vi "CCExtractAllDicomInfoFromFile.vi"(8 "error in (no error)":errorcluster, 11 "filename":string) -> (0 "error out":errorcluster, 2 "Values":string[](array[string]), 3 "VariableName":string[](array[string]))   [LabVIEW 2013, in "main.lvlib" / "ClearCanvasLibrary.lvlib"]
uses:
  ClearCanvasLibrary.lvlib
  C:/Users/Simon/SkyDrive/LabView/2013/DM2020/DICOM/ClearCanvasNewBuild/ClearCanvas.Dicom.dll
  ClearCanvasNewBuild/ClearCanvas.Dicom.dll
panel:
  out "Dump":string
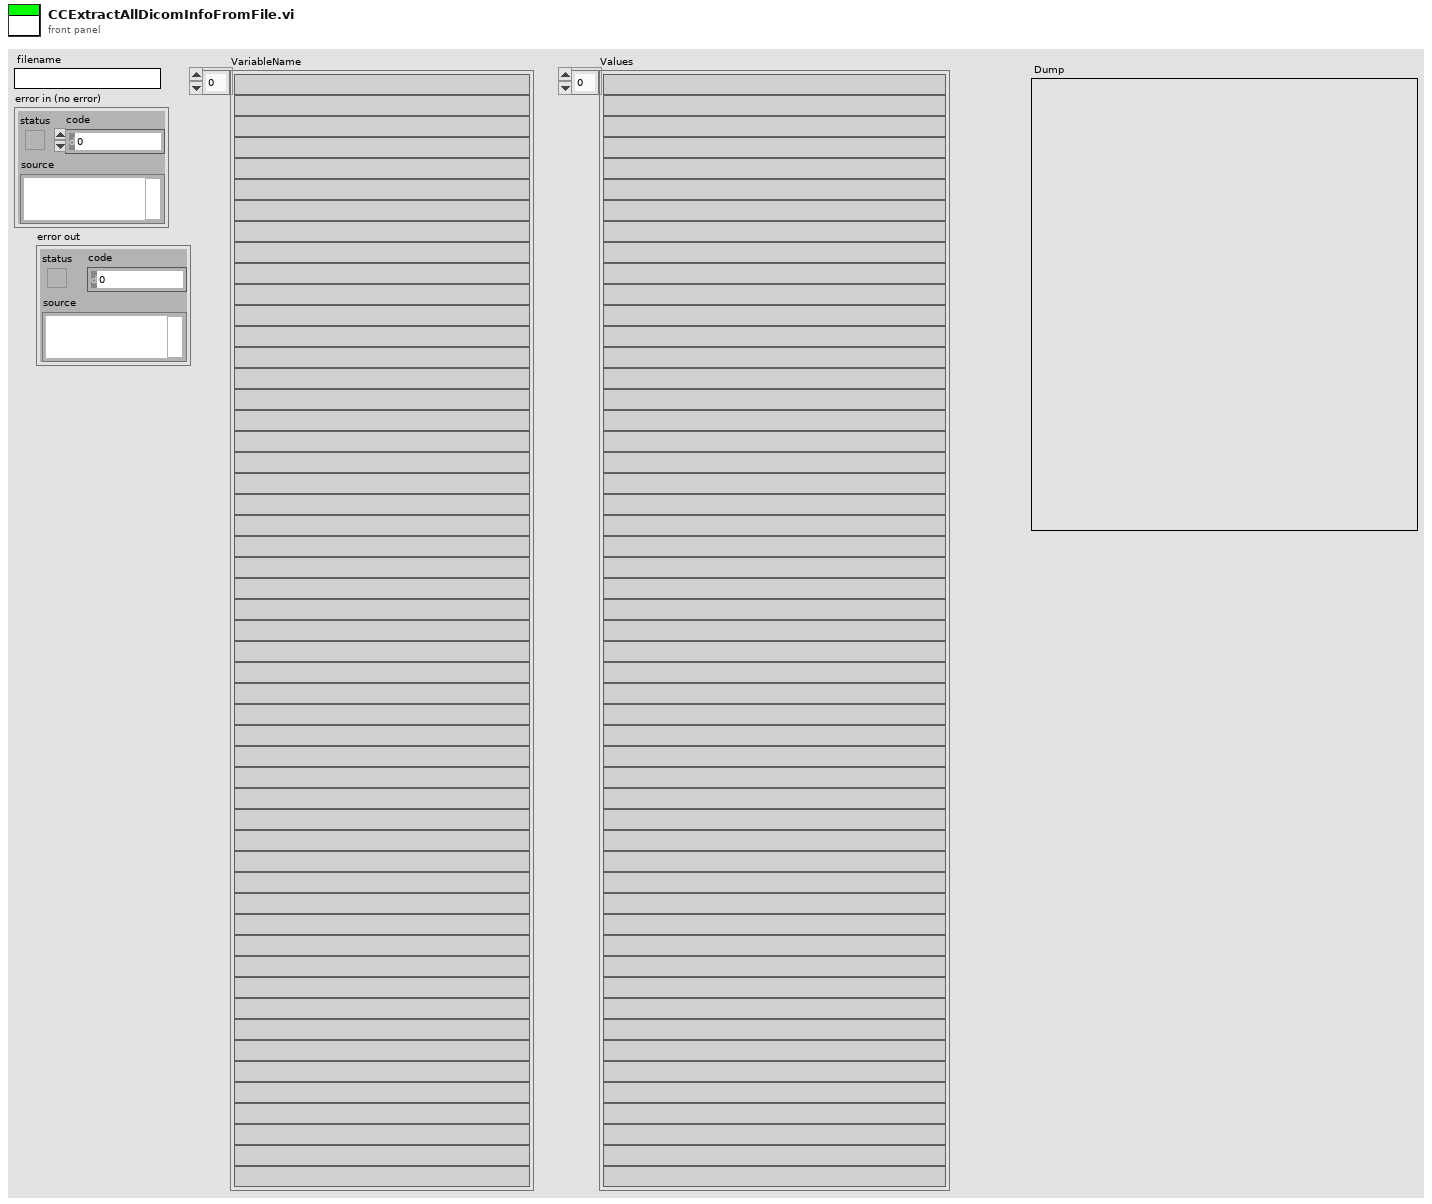
[diagram p1: front panel]
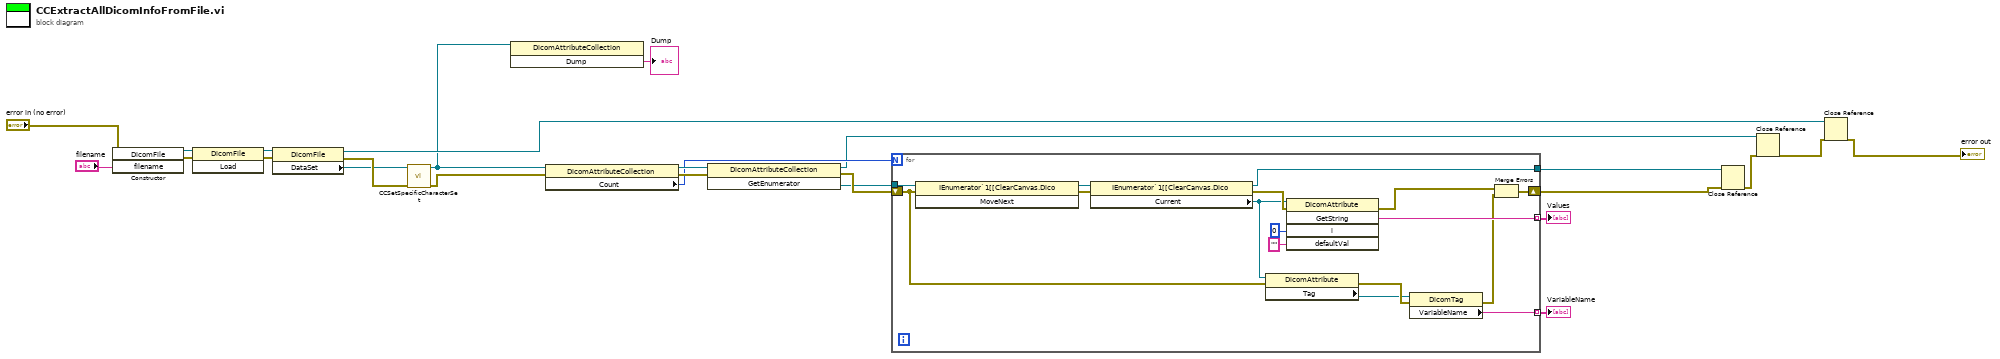
[diagram p0: block diagram]
diagram:
  n1 = constructor class="DicomFile"(error in="error in (no error)", "filename"="filename") -> (reference out=w25:refnum<k24>, error out=w23:errorcluster)  [unwired: 2 in, 2 out]
  n2 = invoke class="DicomFile" method="Load"(reference=w25, error in=w23) -> (reference out=w24:refnum<k24>, error out=w22:errorcluster)  [unwired: 1 in, 1 out]
  n3 = property class="DicomFile"(reference=w24, error in=w22) -> (reference out=w7:refnum<k24>, error out=w4:errorcluster, "DataSet"=w3:refnum<k24>)
  n4 = call "CCSetSpecificCharacterSet.vi"("error in (no error)"=w4, ".NET Refnum in"=w3) -> ("error out"=w2:errorcluster, ".NET Refnum out"=w1:refnum<k24>)  [unwired: 8 in]
  n5 = invoke class="DicomAttributeCollection" method="Dump"(reference=w1) -> ("Dump"=→"Dump":string)  [unwired: 2 in, 2 out]
  n6 = property class="DicomAttributeCollection"(reference=w1, error in=w2) -> (reference out=w18:refnum<k24>, error out=w17:errorcluster, "Count"=w16:i32)
  n7 = invoke class="DicomAttributeCollection" method="GetEnumerator"(reference=w18, error in=w17) -> (reference out=w13:refnum<k24>, error out=w21:errorcluster, "GetEnumerator"=w19:refnum<k24>)  [unwired: 1 in]
  n8 = for {
    N: w16 -> [_]
    tunnel: w19 -> [w41]
    tunnel: [w36] -> w15 mode=indexing
    shift-right: [w31] -> w10
    shift-left: w21 -> [w33]
    tunnel: [w30] -> w11 mode=indexing
    tunnel: [w29] -> w12
    n9 = invoke class="IEnumerator`1[[ClearCanvas.Dico" method="MoveNext"(reference=w41, error in=w33) -> (reference out=w40:refnum<k24>, error out=w39:errorcluster)  [unwired: 1 in, 1 out]
    n10 = property class="IEnumerator`1[[ClearCanvas.Dico"(reference=w40, error in=w39) -> (reference out=w29:refnum<k24>, error out=w35:errorcluster, "Current"=w34:refnum<k24>)
    n11 = property class="DicomAttribute"(reference=w34, error in=w33) -> (error out=w28:errorcluster, "Tag"=w26:refnum<k24>)  [unwired: 1 out]
    n12 = invoke class="DicomAttribute" method="GetString"(reference=w34, error in=w35, "i"=0, "defaultVal"="") -> (error out=w32:errorcluster, "GetString"=w36:string)  [unwired: 1 in, 3 out]
    n13 = property class="DicomTag"(reference=w26, error in=w28) -> (error out=w27:errorcluster, "VariableName"=w30:string)  [unwired: 1 out]
    n14 = Merge Errors(w32, w27) -> (w31:errorcluster)
  }
  "VariableName" <- w11
  "Values" <- w15
  n15 = Close Reference(reference=w12, error in (no error)=w10) -> (error out=w9:errorcluster)
  n16 = Close Reference(reference=w13, error in (no error)=w9) -> (error out=w8:errorcluster)
  n17 = Close Reference(reference=w7, error in (no error)=w8) -> (error out=→"error out":errorcluster)
